vi "Generate Signal.vi"(6 "time (now)":timestamp, 7 "signal type":enum16{"sine", "cosine", "triangle", "square"}(ring), 8 "error in (no error)":errorcluster, 9 "frequency (1)":dbl=1.0 format="%0.2f", 10 "phase (0)":dbl format="%0.2f", 11 "amplitude (1)":dbl=1.0 format="%0.2f") -> (0 "error out":errorcluster, 3 "wave form":dbl format="%0.2f")   [LabVIEW 2019]
doc: "This VI generates a few different types of simulated signals."
uses:
  <vilib>/ptbypt/NI_PtbyPt.lvlib
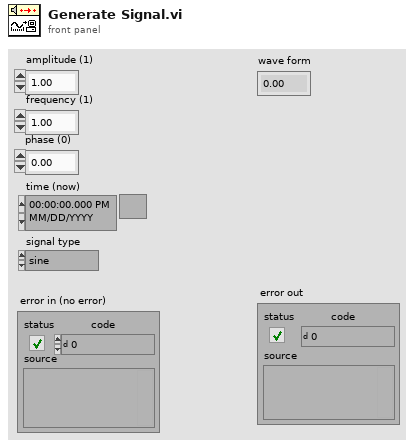
[diagram p1: front panel]
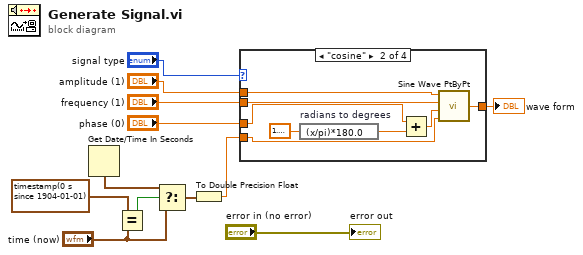
[diagram p0: block diagram]
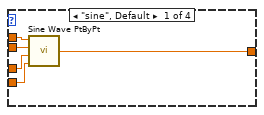
[diagram p2: hidden frame]
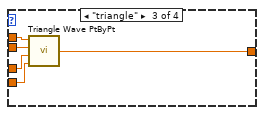
[diagram p3: hidden frame]
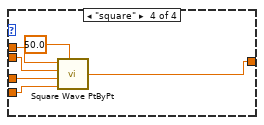
[diagram p4: hidden frame]
diagram:
  n1 = Get Date/Time In Seconds() -> (seconds since 1Jan1904=w4:timestamp)
  n2 = Equal?(x=timestamp(0 s since 1904-01-01) ("time (now)"), y="time (now)") -> (x = y?=w5:bool)
  n3 = Select(t=w4, s=w5, f="time (now)") -> (s? t:f=w2:timestamp)
  n4 = To Double Precision Float(number=w2) -> (double precision float=w6:dbl)
  n5 = case shown="\"cosine\"" "signal type" {
    tunnel: w6 -> [w17 w25 w30 w36]
    tunnel: "phase (0)" -> [w16 w24 w26 w32]
    tunnel: "frequency (1)" -> [w15 w23 w29 w35]
    tunnel: "amplitude (1)" -> [w14 w22 w28 w34]
    tunnel: [w13 w21 w27 w33] -> w9
    frame "sine", Default {
      n6 = call <vilib>:"Sine Wave PtByPt.vi"("time"=w17, "phase"=w16, "frequency"=w15, "amplitude"=w14) -> ("sine wave"=w13:dbl)
    }
    frame "cosine" {
      n7 = expression code="(x/pi)*180.0" "radians to degrees"(1.5707963267948966) -> (w18:dbl)
      n8 = Add(x=w24, y=w18) -> (x+y=w20:dbl)
      n9 = call <vilib>:"Sine Wave PtByPt.vi"("time"=w25, "phase"=w20, "frequency"=w23, "amplitude"=w22) -> ("sine wave"=w21:dbl)
    }
    frame "triangle" {
      n10 = call <vilib>:"Triangle Wave PtByPt.vi"("time"=w30, "phase"=w26, "frequency"=w29, "amplitude"=w28) -> ("triangle wave"=w27:dbl)
    }
    frame "square" {
      n11 = call <vilib>:"Square Wave PtByPt.vi"("amplitude"=w34, "frequency"=w35, "phase"=w32, "time"=w36, "duty cycle (%)"=50.0) -> ("square wave"=w33:dbl)
    }
  }
  "wave form" <- w9
  "error out" <- "error in (no error)"
